vi "LV2 - QueueRef.vi"(7 "Action":enum16{"Set", "Get"}(ring)=enum."Get", 11 "EventLoggerQueue":refnum<queue>) -> (3 "EventLoggerQueue out":refnum<queue>)   [LabVIEW 2019, in "EventLogger.lvlib"]
uses:
  EventLogger.lvlib
  Cluster - MessageCluster.ctl
  Enum - Message.ctl
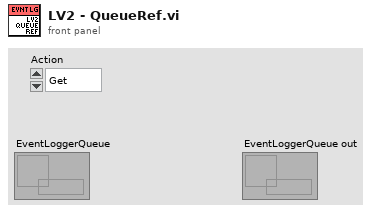
[diagram p1: front panel]
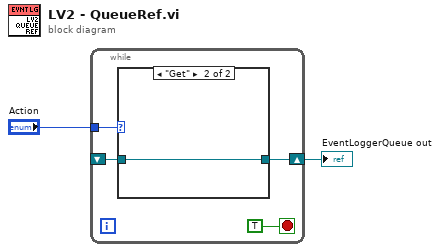
[diagram p0: block diagram]
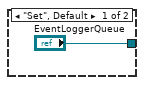
[diagram p2: hidden frame]
diagram:
  n1 = while {
    tunnel: "Action" -> [w6]
    shift-right: [w5] -> w1
    shift-left: _ -> [w4]
    stop <- TRUE stop-if-true
    n2 = case shown="\"Get\"" w6 {
      tunnel: ["EventLoggerQueue" w8] -> w5
      tunnel: w4 -> [_ w8]
      frame "Set", Default {
      }
      frame "Get" {
      }
    }
  }
  "EventLoggerQueue out" <- w1
